vi "LocationSave.vi"(11 "Computer Name":T1) -> (3 "Computer Name Out":T1)   [LabVIEW 2022 SP3]
uses:
  ComputerLocations/ComputerName.ctl
  -ScanSystem/Controls/location.ctl
panel:
  in  "OK Button":bool
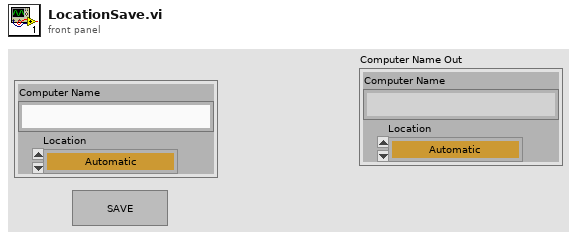
[diagram p1: front panel]
types:
  T1 = typedef "ComputerName.ctl" = cluster{"Computer Name":string, "Location":T2}
  T2 = typedef "location.ctl" = enum16{"Automatic", "WCM Main", "Hawaii", "Columbia MM3000", "Columbia  NI System", "NYU", "RRI 2", "UHI Allen", "CUMC RT", "Chiba", "Stony Brook", "WCM Microscopy", "WCM Aeoretch", "WCM Optics Lab", "WCM Main 2Axis", "WCM Rotation", "WCM SAM SMAC", "SERI GP"}
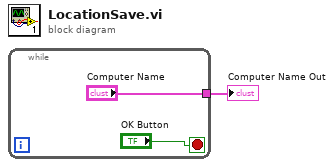
[diagram p0: block diagram]
diagram:
  n1 = while {
    tunnel: ["Computer Name"] -> w1
    stop <- "OK Button" stop-if-true
  }
  "Computer Name Out" <- w1
